vi "Update Displacement.vi"(11 "Motion in":refnum<class "Motion.lvclass">) -> (3 "Motion out":refnum<class "Motion.lvclass">)   [LabVIEW 2021, in "Motion.lvclass"]
uses:
  Motion.lvclass
  Motion.lvclass/Motion.ctl
  Vector 2D/Vector 2D.lvclass
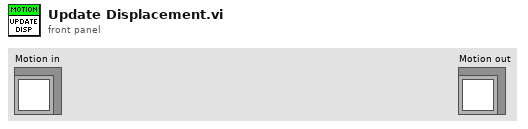
[diagram p1: front panel]
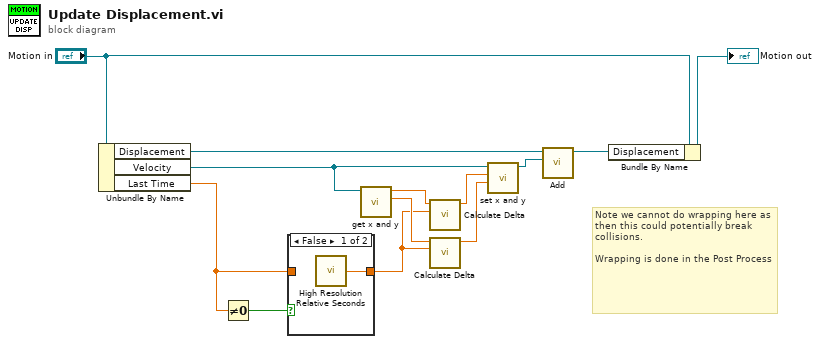
[diagram p0: block diagram]
diagram:
  # "Note we cannot do wrapping here as then this could potentially break collisions.\n\nWrapping is done in the Post Process"
  n1 = Unbundle By Name("Motion in") -> ("Displacement"=w13:refnum<class "Vector 2D.lvclass">, "Velocity"=w9:refnum<class "Vector 2D.lvclass">, "Last Time"=w3:dbl)
  n2 = Not Equal To 0?(x=w3) -> (x != 0?=w4:bool)
  n3 = case shown="False" w4 {
    tunnel: w3 -> [_ w15]
    tunnel: [w14 w15] -> w2
    frame False {
      n4 = call <vilib>:"High Resolution Relative Seconds.vi"() -> ("relative seconds"=w14:dbl)
    }
    frame True {
    }
  }
  n5 = call "get x and y.vi"("Vector 2D in"=w9) -> ("y"=w6:sgl, "x"=w8:sgl)  [unwired: 9 in]
  n6 = call "Calculate Delta.vi"("Last Time"=w2, "Property"=w8) -> ("Delta"=w7:sgl)  [unwired: 9 in]
  n7 = call "Calculate Delta.vi"("Last Time"=w2, "Property"=w6) -> ("Delta"=w5:sgl)  [unwired: 9 in]
  n8 = call "set x and y.vi"("y"=w5, "x"=w7, "Vector 2D in"=w9) -> ("Vector 2D out"=w10:refnum<class "Vector 2D.lvclass">)  [unwired: 8 in]
  n9 = call "Add.vi"("Vector 2D B in"=w10, "Vector 2D in"=w13) -> ("Vector 2D out"=w1:refnum<class "Vector 2D.lvclass">)  [unwired: 9 in]
  n10 = Bundle By Name(cluster="Motion in", "Displacement"=w1) -> (→"Motion out":refnum<class "Motion.lvclass">)
